vi "FPGA Simple PWM U8.vi"(7 "PWM Enabled?":bool, 10 "Low Count":u8, 11 "High Count":u8) -> (3 "PWM Output":bool)   [LabVIEW 2015]
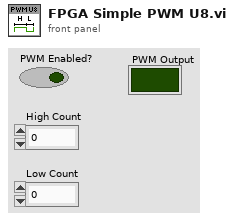
[diagram p1: front panel]
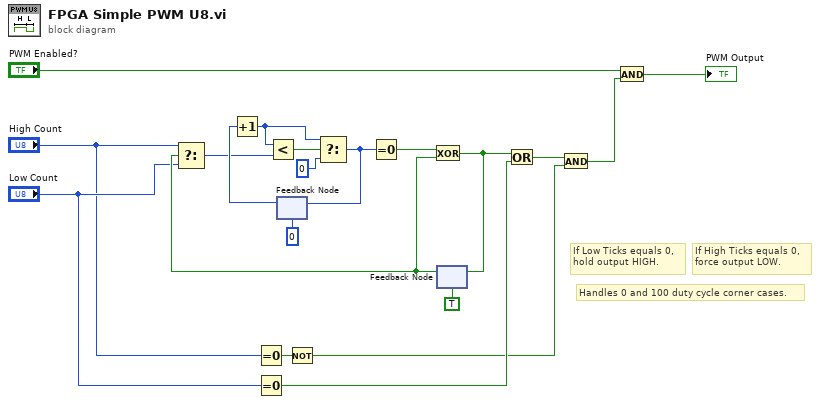
[diagram p0: block diagram]
diagram:
  # "Handles 0 and 100 duty cycle corner cases."
  # "If High Ticks equals 0,\nforce output LOW."
  # "If Low Ticks equals 0,\nhold output HIGH."
  n1 = Equal To 0?(x="High Count") -> (x = 0?=w7:bool)
  n2 = Equal To 0?(x="Low Count") -> (x = 0?=w4:bool)
  n3 = feedback #1(u8 0 ("High Ticks")) -> (w13:u8)
  n4 = Increment(x=w13) -> (x+1=w12:u8)
  n5 = Not(x=w7) -> (.not. x?=w2:bool)
  n6 = feedback #2(TRUE) -> (w11:bool)
  n7 = Select(t="High Count", s=w11, f="Low Count") -> (s? t:f=w10:u8)
  n8 = Less?(x=w12, y=w10) -> (x < y?=w18:bool)
  n9 = Select(t=w12, s=w18, f=u8 0) -> (s? t:f=w20:u8)
  n10 = feedback-in #1(w20) -> ()
  n11 = Equal To 0?(x=w20) -> (x = 0?=w8:bool)
  n12 = Exclusive Or(1:w11, 2:w8) -> (0:w5:bool)
  n13 = feedback-in #2(w5) -> ()
  n14 = Or(x=w5, y=w4) -> (x .or. y?=w3:bool)
  n15 = And(x=w3, y=w2) -> (x .and. y?=w1:bool)
  n16 = And(x="PWM Enabled?", y=w1) -> (x .and. y?=→"PWM Output":bool)
